vi "New.vi"(8 "error in (no error)":errorcluster, 10 "Parent":refnum<class "Config Element.lvclass">, 11 "System Name":string) -> (0 "error out":errorcluster, 2 "Config Element":refnum<class "Config Element.lvclass">, 3 "System out":refnum<class "System.lvclass">)   [LabVIEW 2020, in "VolatusConfig.lvlib" / "System.lvclass"]
uses:
  System.lvclass
  C:/dev/lv20CE/relink/lv-volatus/VolatusConfig/VolatusConfigElement/VolatusConfigElement.lvclass
  lv-cdm/CDM-Config/Config Element/Config Element.lvclass
  lv-cdm/CDM-Config/Value Type.ctl
  Meta Type.ctl
  VolatusConfigElement/VolatusConfigElement.lvclass
  lv-cdm/CDM-Config/CDM-Config.lvlib
  VolatusConfig.lvlib
  SensorList/SensorList.lvclass
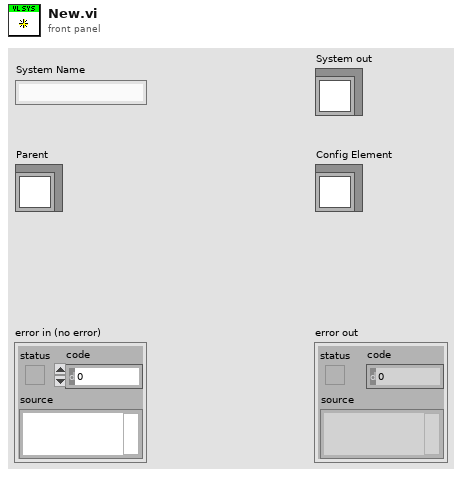
[diagram p1: front panel]
types:
  T1 = typedef "VolatusConfig.lvlib/Meta Type.ctl" = enum16{"UNKNOWN", "VL_System", "VL_Cluster", "VL_Node", "VL_Task", "VL_Group", "VL_Channel", "VL_Task_List", "VL_Scaling", "VL_Sensor", "VL_Sensor_List", "VL_Scale"}
  T2 = typedef "CDM-Config.lvlib/Value Type.ctl" = enum16{"String", "Number", "Bool", "Object", "Array"}
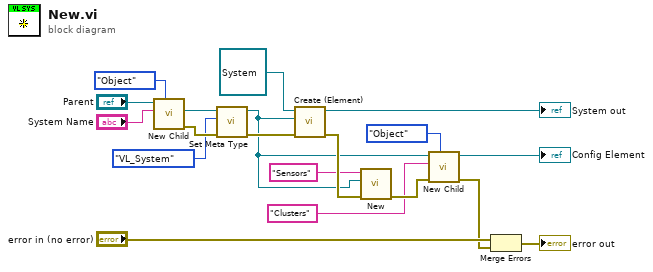
[diagram p0: block diagram]
diagram:
  n1 = call "New Child.vi"("Value Type (Object)"=Value_Type."Object" ("Value Type (String)"), "Child Name"="System Name", "Config Element in"="Parent") -> ("error out"=w12:errorcluster, "New Child"=w4:refnum<class "Config Element.lvclass">)  [unwired: 6 in, 1 out]
  n2 = call "Set Meta Type.vi"("error in (no error)"=w12, "Meta Type"=Meta_Type."VL_System", "Element In"=w4) -> ("error out"=w5:errorcluster, "Element"=w3:refnum<class "Config Element.lvclass">)  [unwired: 7 in]
  n3 = call "Create (Element).vi"("error in (no error)"=w5, "Element"=w3, "VolatusConfigElement in"=refnum<class "System.lvclass"> refnum ("System in")) -> ("error out"=w18:errorcluster, "VolatusConfigElement out"=→"System out":refnum<class "System.lvclass">)  [unwired: 7 in]
  n4 = call "New.vi"("error in (no error)"=w18, "Parent"=w3, "Name"="Sensors" ("System Name")) -> ("error out"=w19:errorcluster)  [unwired: 7 in, 1 out]
  n5 = call "New Child.vi"("Value Type (Object)"=Value_Type."Object" ("Value Type (String)"), "error in (no error)"=w19, "Child Name"="Clusters" ("System Name"), "Config Element in"=w3) -> ("error out"=w6:errorcluster, "Config Element out"=→"Config Element":refnum<class "Config Element.lvclass">)  [unwired: 5 in, 1 out]
  n6 = Merge Errors("error in (no error)", w6) -> (→"error out":errorcluster)
